vi "SVL Set dB Reference (variant).vi"(8 "error in (no error)":errorcluster, 10 "dB reference [EU]":dbl=1.0 format="%^.1e", 11 "attributes in":variant) -> (0 "error out":errorcluster, 3 "attributes out":variant)   [LabVIEW 2017]
doc: "Sets the specified <B>dB reference [EU]</B> as an attribute in the <B>scaled signal out [EU]</B> waveform. <B>dB reference [EU]</B> is used for all downstream conversions to dB. Wire data to the <B>scaled signal in [EU]</B> input to determine the polymorphic instance to use or manually select the instance."
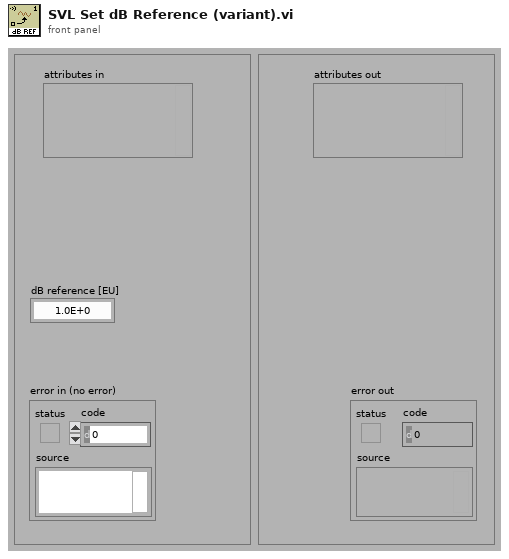
[diagram p1: front panel]
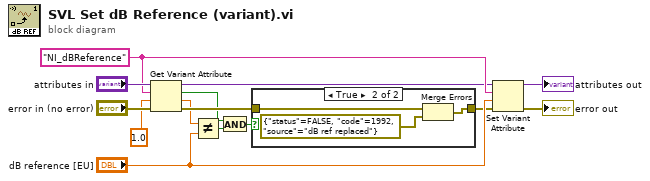
[diagram p0: block diagram]
diagram:
  w10 = "NI_dBReference" ("name")
  n1 = Get Variant Attribute(Variant="attributes in", name=w10, default value (empty Variant)=1.0 ("dB reference [EU]"), error in="error in (no error)") -> (duplicate Variant=w6:variant, found=w4:bool, value=w3:dbl, error out=w8:errorcluster)
  n2 = Not Equal?(x=w3, y="dB reference [EU]") -> (x != y?=w2:bool)
  n3 = And(x=w4, y=w2) -> (x .and. y?=w1:bool)
  n4 = case shown="True" w1 {
    tunnel: w8 -> [w15 w18]
    tunnel: [w15 w17] -> w7
    frame False {
    }
    frame True {
      n5 = Merge Errors(w18, errorcluster {"status"=FALSE, "code"=1992, "source"="dB ref replaced"} ("error out")) -> (w17:errorcluster)
    }
  }
  n6 = Set Variant Attribute(Variant=w6, name=w10, value="dB reference [EU]", error in=w7) -> (Variant out=→"attributes out":variant, error out=→"error out":errorcluster)  [unwired: 1 out]
